vi "Set and Get Mlistbox Size.vi"(7 "Mode":T2, 8 "错误输入":errorcluster, 10 "Size In":T1 caption="大小", 11 "Mlistbox Ref":refnum<vi>) -> (0 "错误输出":errorcluster, 2 "Size Out":T1 caption="大小", 3 "Mlistbox Ref Dup":refnum<vi>)   [LabVIEW 2012, in "Mlistbox Tools.lvlib"]
uses:
  Mlistbox Tools.lvlib
  ListBox/Custom Type/Read and Write Mode.ctl
  <vilib>/Utility/miscctls.llb/LVBoundsTypeDef.ctl
  ListBox/Listbox Tool.lvlib
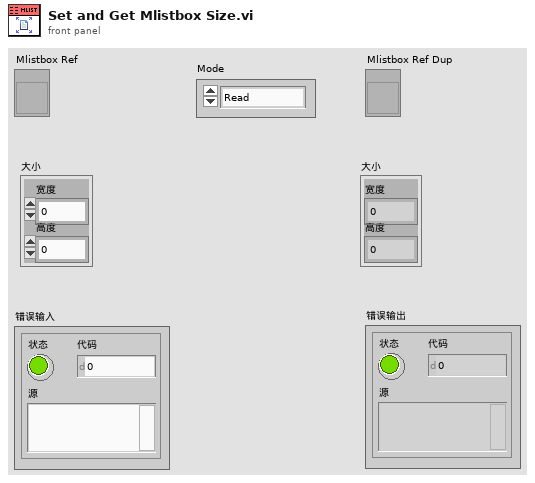
[diagram p1: front panel]
types:
  T1 = typedef "LVBoundsTypeDef.ctl" = cluster{"Width":u32, "Height":u32}
  T2 = typedef "Listbox Tool.lvlib/Read and Write Mode.ctl" = enum16{"Read", "Write"}
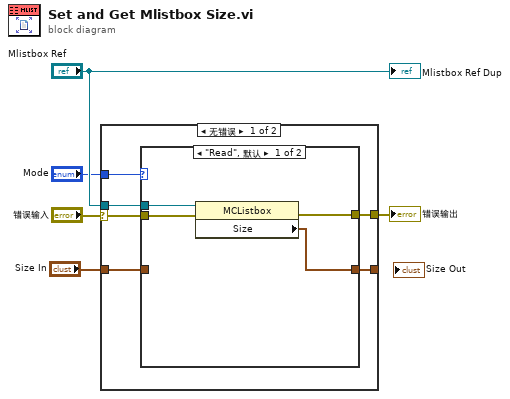
[diagram p0: block diagram]
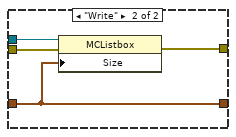
[diagram p2: hidden frame]
diagram:
  n1 = case shown="无错误" "错误输入" {
    selector: "错误输入" -> [w9 w20]
    tunnel: [w7 w20] -> w4
    tunnel: "Mlistbox Ref" -> [w10 _]
    tunnel: "Mode" -> [w11 _]
    tunnel: [w8 _] -> _
    tunnel: "Size In" -> [w6 _]
    frame No Error {
      n2 = case shown="\"Read\", 默认" w11 {
        tunnel: w10 -> [w15 w19]
        tunnel: w9 -> [w14 w18]
        tunnel: [w13 w16] -> w8
        tunnel: [w12 w17] -> w7
        tunnel: w6 -> [_ w16]
        frame "Read", Default {
          n3 = property class="MCListbox"(reference=w15, error in=w14) -> (error out=w12:errorcluster, "Size"=w13:T1)  [unwired: 1 out]
        }
        frame "Write" {
          n4 = property class="MCListbox"(reference=w19, error in=w18, "Size"=w16) -> (error out=w17:errorcluster)  [unwired: 1 out]
        }
      }
    }
    frame Error {
    }
  }
  "错误输出" <- w4
  "Mlistbox Ref Dup" <- "Mlistbox Ref"
